vi "Inficon - Set max power.vi"(8 "Error In":errorcluster, 10 "Max Power":dbl=0.1 min=0.0 max=100.0 step=0.1 format="%.;%.1f", 11 "COM in":refnum<visa-resource-name>) -> (0 "Error Out":errorcluster, 3 "COM out":refnum<visa-resource-name>)   [LabVIEW 2014]
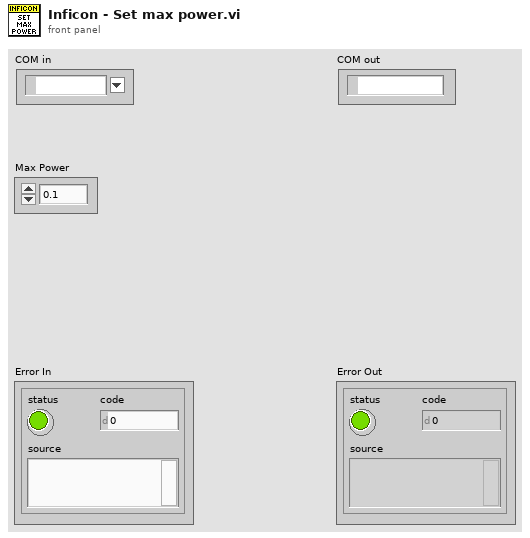
[diagram p1: front panel]
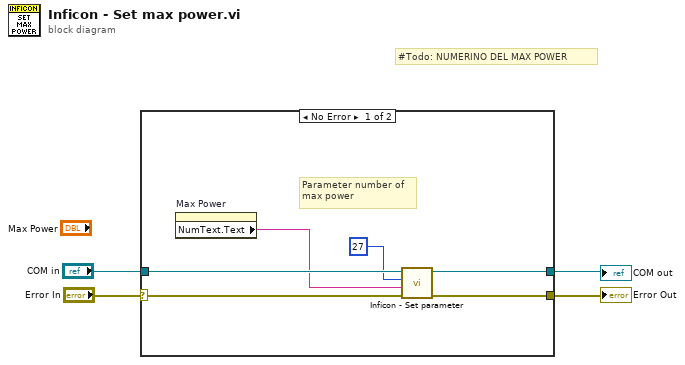
[diagram p0: block diagram]
diagram:
  # "#Todo: NUMERINO DEL MAX POWER"
  n1 = case shown="No Error" "Error In" {
    selector: "Error In" -> [w10 w11]
    tunnel: [w9 w11] -> w3
    tunnel: "COM in" -> [w8 w12]
    tunnel: [w7 w12] -> w1
    frame No Error {
      # "Parameter number of\nmax power"
      n2 = property on="Max Power" class="DigNum (strict)"() -> ("NumText.Text"=w5:string)  [unwired: 2 in, 2 out]
      n3 = call "Inficon - Set parameter.vi"("Error In"=w10, "Param value"=w5, "Param number"=u8 27, "COM in"=w8) -> ("Error Out"=w9:errorcluster, "COM out"=w7:refnum<visa-resource-name>)  [unwired: 6 in]
    }
    frame Error {
    }
  }
  "Error Out" <- w3
  "COM out" <- w1
